vi "Unreserve GPIO.vi"(8 "error in (no error)":errorcluster, 10 "GPIO #":T1=-1, 11 "Session in":refnum<class "Session.lvclass">) -> (0 "error out":errorcluster, 3 "Session out":refnum<class "Session.lvclass">)   [LabVIEW 2024, in "CTI.lvlib" / "Session.lvclass"]
uses:
  Session.lvclass
  GPIO Number.ctl
  Session.lvclass/Session.ctl
  6bf7663a-2450-4584-aa50-52eb657dd743.vi
  8b3d9e06-e34d-461d-a711-d0ed6439524f.vi
  8b3d9e06-e34d-461d-a711-d0ed6439524f.vi/685f7f19-b444-4620-8f66-e6e2ddd64bb8.vi
  GPIO/GPIO.lvclass
  C:/Users/nkirchne/Documents/~SANDBOX/Electronics Workflow/build/ForPort/CTI/Resource/Resource.lvclass
  Generate Error.vi
  Resource/Resource.lvclass
  CTI.lvlib
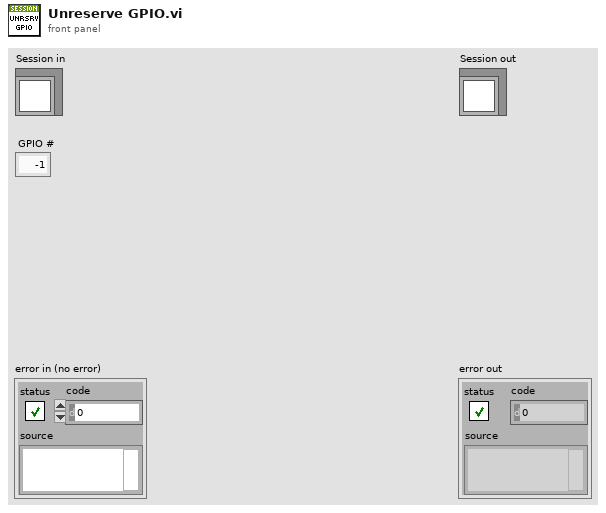
[diagram p1: front panel]
types:
  T1 = typedef "CTI.lvlib/GPIO Number.ctl" = i8
  T2 = typedef "CTI.lvlib/Session.lvclass/Resources.ctl" = cluster{"GPIO":map{T1, refnum<class "GPIO.lvclass">}, "AI":map{T3, refnum<class "AI.lvclass">}, "PWM":map{T1, refnum<class "PWM.lvclass">}, "UART":map{T4, refnum<class "UART.lvclass">}, "I2C":map{T5, refnum<class "I2C.lvclass">}, "SPI":map{T6, refnum<class "SPI.lvclass">}, "SPI CS":map{T1, refnum<class "SPI CS.lvclass">}}
  T3 = typedef "CTI.lvlib/ADC Number.ctl" = i8
  T4 = typedef "CTI.lvlib/UART Number.ctl" = i8
  T5 = typedef "CTI.lvlib/I2C Number.ctl" = i8
  T6 = typedef "CTI.lvlib/SPI Number.ctl" = i8
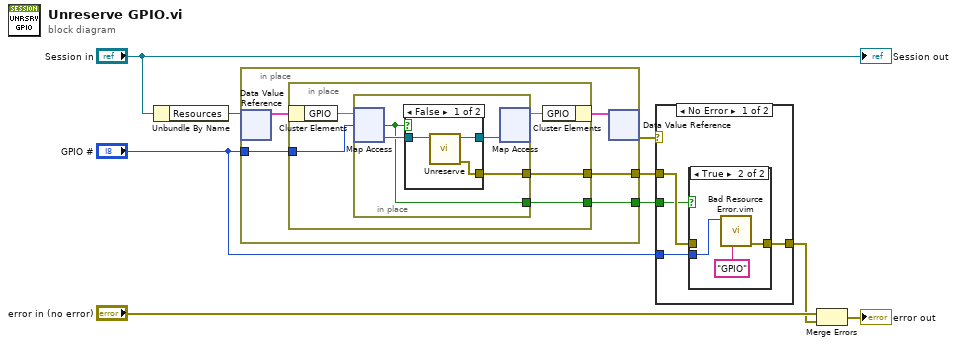
[diagram p0: block diagram]
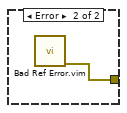
[diagram p3: hidden frame]
diagram:
  n1 = Unbundle By Name("Session in") -> ("Resources"=w9:refnum<data-value>)
  n2 = in-place {
    in-place-border: "GPIO #" -> [w14]
    in-place-border: [w13] -> w4
    in-place-border: [w12] -> w7
    n3 = in-place-dvr #1(w9) -> (w10:T2)  [unwired: 1 out]
    n4 = in-place {
      in-place-border: w14 -> [w18]
      in-place-border: [w17] -> w13
      in-place-border: [w16] -> w12
      n5 = in-place-cluster #2(w10) -> ("GPIO"=w19:map{T1, refnum<class "GPIO.lvclass">})
      n6 = in-place {
        in-place-border: [w22] -> w16
        in-place-border: [w21] -> w17
        n7 = in-place-map #3(w19, w18) -> (w23:refnum<class "GPIO.lvclass">, w21:bool)  [unwired: 1 in]
        n8 = case shown="False" w21 {
          tunnel: w23 -> [w26 w27]
          tunnel: [w25 w27] -> w20
          tunnel: [w24 _] -> w22
          frame False {
            n9 = call "Unreserve.vi"("Resource in"=w26) -> ("error out"=w24:errorcluster, "Resource out"=w25:refnum<class "GPIO.lvclass">)  [unwired: 9 in]
          }
          frame True {
          }
        }
        n10 = in-place-map #3(w20) -> (w15:map{T1, refnum<class "GPIO.lvclass">})  [unwired: 1 in, 2 out]
      }
      n11 = in-place-cluster #2("GPIO"=w15) -> (w11:T2)
    }
    n12 = in-place-dvr #1(w11) -> (w6:errorcluster)  [unwired: 1 out]
  }
  n13 = case shown="No Error" w6 {
    tunnel: w7 -> [w31 _]
    tunnel: w4 -> [w30 _]
    tunnel: [w29 w36] -> w1
    tunnel: "GPIO #" -> [w28 _]
    frame No Error {
      n14 = case shown="True" w30 {
        tunnel: w31 -> [w32 _]
        tunnel: [w32 w35] -> w29
        tunnel: w28 -> [_ w34]
        frame False {
        }
        frame True {
          n15 = call "Bad Resource Error.vim"("Resource Type"="GPIO", "Res #"=w34) -> ("error out"=w35:errorcluster)  [unwired: 9 in]
        }
      }
    }
    frame Error {
      n16 = call "Bad Ref Error.vim"() -> ("error out"=w36:errorcluster)  [unwired: 10 in, 1 out]
    }
  }
  n17 = Merge Errors("error in (no error)", w1) -> (→"error out":errorcluster)
  "Session out" <- "Session in"
